vi "Accel. Limit.vi"(10 "Max Change":dbl=0.2, 11 "Drive Controls":T1) -> (3 "Drive Controls 2":T1)   [LabVIEW 2014]
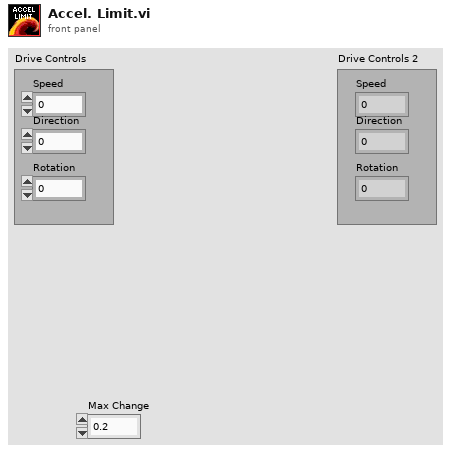
[diagram p1: front panel]
types:
  T1 = cluster{"Speed":dbl, "Direction":dbl, "Rotation":dbl}
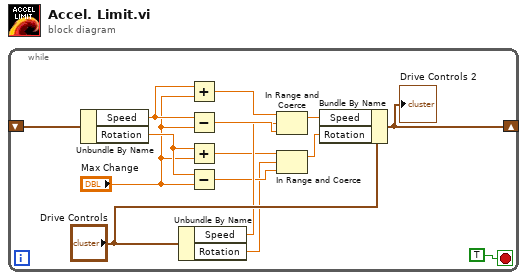
[diagram p0: block diagram]
diagram:
  n1 = while {
    shift-right: [w12] -> _
    shift-left: _ -> [w11]
    stop <- TRUE stop-if-true
    n2 = Unbundle By Name(w11) -> ("Speed"=w8:dbl, "Rotation"=w3:dbl)
    n3 = Unbundle By Name("Drive Controls") -> ("Speed"=w7:dbl, "Rotation"=w4:dbl)
    n4 = Add(x=w8, y="Max Change") -> (x+y=w15:dbl)
    n5 = Subtract(x=w8, y="Max Change") -> (x-y=w9:dbl)
    n6 = Add(x=w3, y="Max Change") -> (x+y=w5:dbl)
    n7 = Subtract(x=w3, y="Max Change") -> (x-y=w6:dbl)
    n8 = In Range and Coerce(upper limit=w15, x=w7, lower limit=w9) -> (coerced(x)=w13:dbl)  [unwired: 1 out]
    n9 = In Range and Coerce(upper limit=w5, x=w4, lower limit=w6) -> (coerced(x)=w1:dbl)  [unwired: 1 out]
    n10 = Bundle By Name(cluster="Drive Controls", "Speed"=w13, "Rotation"=w1) -> (w12:T1)
    "Drive Controls 2" <- w12
  }
